vi "CheckNodeName.vi"(3 "node":string) -> (0 "error out":errorcluster, 1 "Node":cluster{"name":string, "Port":u16})   [LabVIEW 2018]
doc: "Checks the node name and opens a new node if the name does not exist"
uses:
  <userlib>/ROS for LabVIEW Software/ROS/Code/SubVIs/_ROSControl.ctl
  <userlib>/ROS for LabVIEW Software/ROS/Code/SubVIs/_ROSDirection.ctl
  <userlib>/ROS for LabVIEW Software/ROS/Code/_ROSDefinition.vi
panel:
  out "compare":string
  out "checked":string[](array[string])
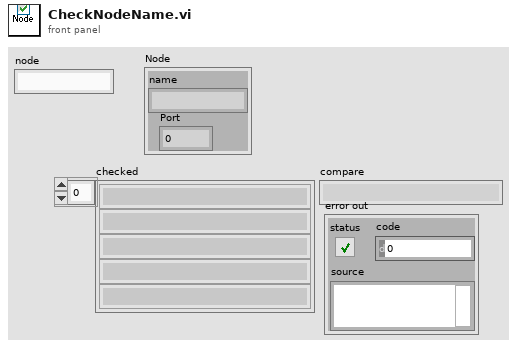
[diagram p1: front panel]
types:
  T1 = typedef "_ROSControl.ctl" = cluster{"topic port":u16, "Node":string, "topic":string, "type":string, "node port":u16, "error ":errorcluster, "Direction":T2, "Update (ms)":u16, "FIFO size":u16}
  T2 = typedef "_ROSDirection.ctl" = enum16{"Node", "Publisher", "Subscriber", "ServiceClient", "ServiceProvider"}
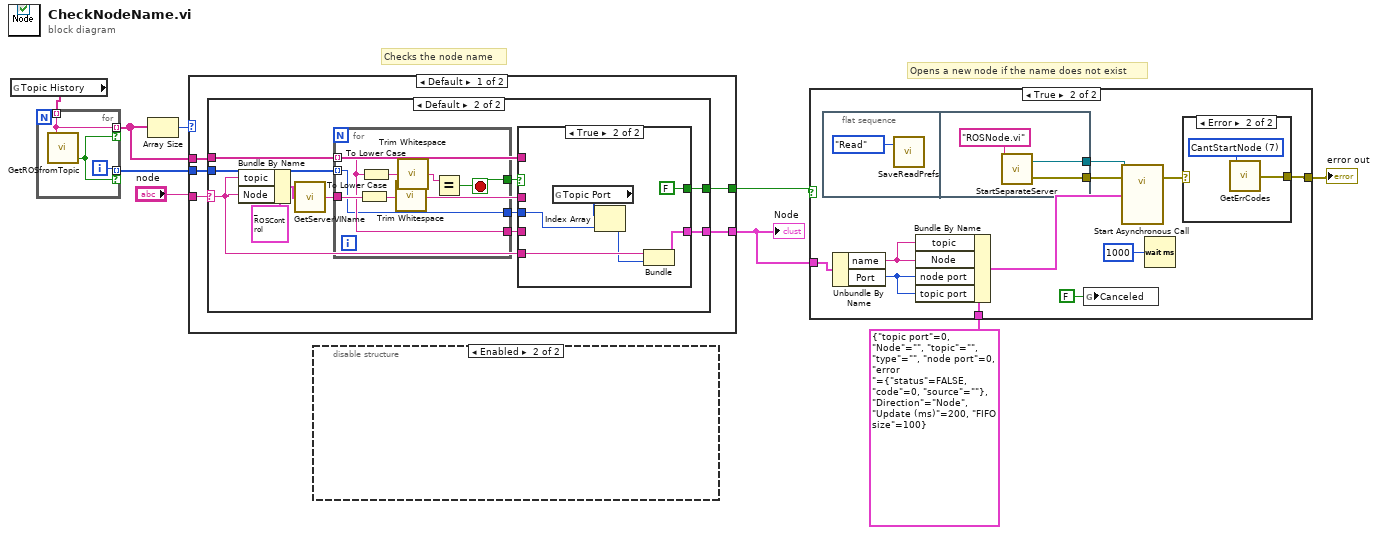
[diagram p0: block diagram]
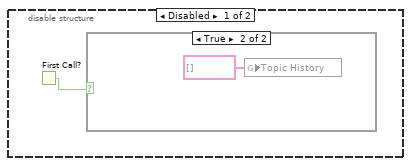
[diagram p2: hidden frame]
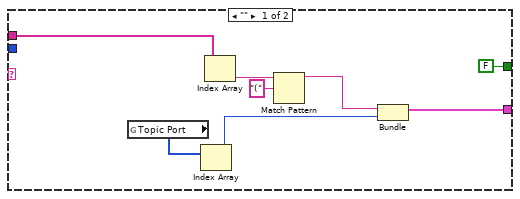
[diagram p4: hidden frame]
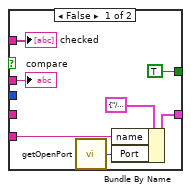
[diagram p5: hidden frame]
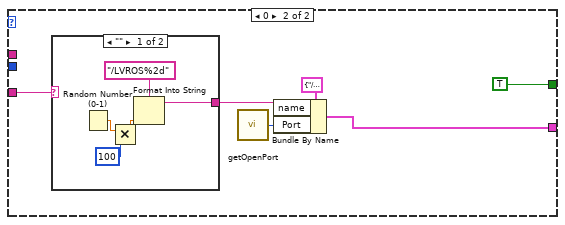
[diagram p6: hidden frame]
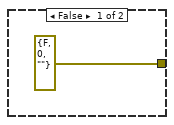
[diagram p8: hidden frame]
diagram:
  # "Opens a new node if the name does not exist"
  # "Checks the node name"
  n1 = global read "_ROSDefinition.vi" "Topic History"() -> (w4:string[])
  n2 = for {
    tunnel: w4 -> [w12] mode=indexing
    tunnel: [w12] -> w3 mode=indexing if=w10
    tunnel: [w11] -> w2 mode=indexing if=w10
    i -> [w11]
    n3 = call <userlib>:"GetROSfromTopic.vi"("Topic"=w12) -> ("Node?"=w10:bool)  [unwired: 1 in, 2 out]
  }
  n4 = Array Size(array=w3) -> (size(s)=w6:i32)
  n5 = case shown="Default" w6 {
    tunnel: "node" -> [w17 w63]
    tunnel: [w15 TRUE] -> w9
    tunnel: [w14 w58] -> w8
    tunnel: w3 -> [w16 _]
    tunnel: w2 -> [w13 _]
    frame Default {
      n6 = case shown="Default" w17 {
        selector: w17 -> [_ w26]
        tunnel: [w22 w36] -> w14
        tunnel: w16 -> [w18 w35]
        tunnel: [FALSE w32] -> w15
        tunnel: w13 -> [_ w27]
        frame "" {
          n7 = global read "_ROSDefinition.vi" "Topic Port"() -> (w24:u16[])
          n8 = Index Array(array=w24) -> (element=w23:u16)  [unwired: 1 in]
          n9 = Index Array(array=w18) -> (element=w20:string)  [unwired: 1 in]
          n10 = Match Pattern(string=w20, regular expression="(") -> (before substring=w19:string)  [unwired: 1 in, 3 out]
          n11 = Bundle("ROS Master"=w19, "Ports"=w23) -> (w22:cluster{"ROS Master":string, "Ports":u16})  [unwired: 1 in]
        }
        frame Default {
          n12 = Bundle By Name(cluster=T1 {"topic port"=0, "Node"="", "topic"="", "type"="", "node port"=0, "error "={"status"=FALSE, "code"=0, "source"=""}, "Direction"=enum."Node", "Update (ms)"=200, "FIFO size"=100} ("ROS"), "topic"=w26, "Node"=w26) -> (w29:T1)
          n13 = call <userlib>:"GetServerVIName.vi"("ROS"=w29) -> ("vi name"=w28:string)
          n14 = for {
            tunnel: w28 -> [w53]
            tunnel: [w55] -> w33
            tunnel: [w51] -> w34
            tunnel: w35 -> [w51] mode=indexing
            tunnel: [w50] -> w31
            tunnel: w27 -> [w50] mode=indexing
            stop <- w55 stop-if-true
            n15 = To Lower Case(string=w53) -> (all lower case string=w54:string)
            n16 = To Lower Case(string=w51) -> (all lower case string=w57:string)
            n17 = call <vilib>:"Trim Whitespace.vi"("string"=w54) -> ("trimmed string"=w52:string)  [unwired: 1 in]
            n18 = call <vilib>:"Trim Whitespace.vi"("string"=w57) -> ("trimmed string"=w56:string)  [unwired: 1 in]
            n19 = Equal?(x=w56, y=w52) -> (x = y?=w55:bool)
          }
          n20 = case shown="True" w33 {
            tunnel: [w42 w44] -> w36
            tunnel: w34 -> [_ _]
            tunnel: w35 -> [w38 _]
            tunnel: w26 -> [w43 w48]
            tunnel: [TRUE FALSE] -> w32
            tunnel: w31 -> [_ w47]
            tunnel: w28 -> [w37 _]
            frame False {
              n21 = call <userlib>:"getOpenPort.vi"() -> ("port"=w41:u16)
              n22 = Bundle By Name(cluster=cluster{"name":string, "Port":u16} {"name"="/LVROS", "Port"=0} ("Node"), "name"=w43, "Port"=w41) -> (w42:cluster{"name":string, "Port":u16})
              "checked" <- w38
              "compare" <- w37
            }
            frame True {
              n23 = global read "_ROSDefinition.vi" "Topic Port"() -> (w46:u16[])
              n24 = Index Array(array=w46, index=w47) -> (element=w45:u16)
              n25 = Bundle(w48, "Ports"=w45) -> (w44:cluster{string, "Ports":u16})  [unwired: 1 in]
            }
          }
        }
      }
    }
    frame 0 {
      n26 = case shown="\"\"" w63 {
        selector: w63 -> [_ w69]
        tunnel: [w64 w69] -> w60
        frame "" {
          n27 = Random Number (0-1)() -> (number: 0 to 1=w67:dbl)
          n28 = Multiply(x=w67, y=100) -> (x*y=w66:dbl)
          n29 = Format Into String(format string="/LVROS%2d" ("name"), w66) -> (resulting string=w64:string)  [unwired: 2 in, 1 out]
        }
        frame Default {
        }
      }
      n30 = call <userlib>:"getOpenPort.vi"() -> ("port"=w61:u16)
      n31 = Bundle By Name(cluster=cluster{"name":string, "Port":u16} {"name"="/LVROS", "Port"=0} ("Node"), "name"=w60, "Port"=w61) -> (w58:cluster{"name":string, "Port":u16})
    }
  }
  "Node" <- w8
  n32 = disable-structure shown="Enabled" {
    frame Disabled {
      n33 = First Call?() -> (First Call?: T/F=w70:bool)
      n34 = case shown="True" w70 {
        frame False {
        }
        frame True {
          n35 = global write "_ROSDefinition.vi" "Topic History"(string[] [] ("Topic History")) -> ()
        }
      }
    }
    frame Enabled {
    }
  }
  n36 = case shown="True" w9 {
    tunnel: w8 -> [_ w83]
    tunnel: T1 {"topic port"=0, "Node"="", "topic"="", "type"="", "node port"=0, "error "={"status"=FALSE, "code"=0, "source"=""}, "Direction"=enum."Node", "Update (ms)"=200, "FIFO size"=100} ("ROS") -> [_ w82]
    tunnel: [errorcluster {"status"=FALSE, "code"=0, "source"=""} ("error out") w73] -> w1
    frame False {
    }
    frame True {
      n37 = flat-sequence {
        tunnel: [w89] -> w79
        tunnel: [w88] -> w78
        frame #0 {
          n38 = call <userlib>:"SaveReadPrefs.vi"("Task"=enum16{"Read", "Save"}."Read") -> ()  [unwired: 2 in, 1 out]
        }
        frame #1 {
          n39 = call <userlib>:"StartSeparateServer.vi"("Server"="ROSNode.vi") -> ("error out"=w89:errorcluster, "Ref out"=w88:refnum<vi>)  [unwired: 1 in]
        }
      }
      n40 = Unbundle By Name(w83) -> ("name"=w81:string, "Port"=w80:u16)
      n41 = Bundle By Name(cluster=w82, "topic"=w81, "Node"=w81, "node port"=w80, "topic port"=w80) -> (w77:T1)
      n42 = global write "_ROSDefinition.vi" "Canceled"(FALSE ("Canceled")) -> ()
      n43 = call-by-ref "Start Asynchronous Call"(reference=w78, error in=w79, "ROS"=w77) -> (error out=w74:errorcluster)  [unwired: 3 in, 1 out]
      n44 = Wait (ms)(milliseconds to wait=u32 1000) -> ()  [unwired: 1 out]
      n45 = case shown="Error" w74 {
        selector: w74 -> [w84 _]
        tunnel: [w84 w85] -> w73
        frame No Error {
        }
        frame Error {
          w86 = u16 7 items=["TopicReadTimeout", "Read=SS", "GetQueueErr", "NoMaster", "Write=PS", "Unparse", "ServiceReply", "CantStartNode"] ("Error")
          n46 = call <userlib>:"GetErrCodes.vi"("Error"=w86) -> ("Error"=w85:errorcluster)  [unwired: 1 in]
        }
      }
    }
  }
  "error out" <- w1
